vi "Panel Is Dead.vi"(8 "error in (no error)":errorcluster, 11 "Panel Control_Ref in":refnum<class "Panel Controller.lvclass">) -> (0 "error out":errorcluster, 3 "Panel Control_Ref out":refnum<class "Panel Controller.lvclass">)   [LabVIEW 2015, in "Panel Controller.lvclass"]
uses:
  Panel Controller.lvclass
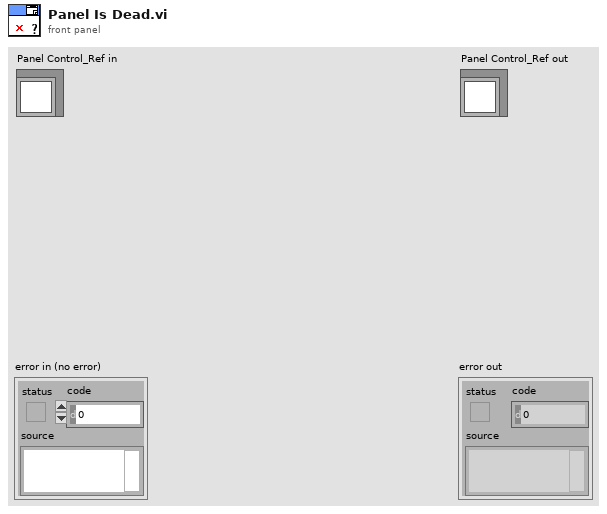
[diagram p1: front panel]
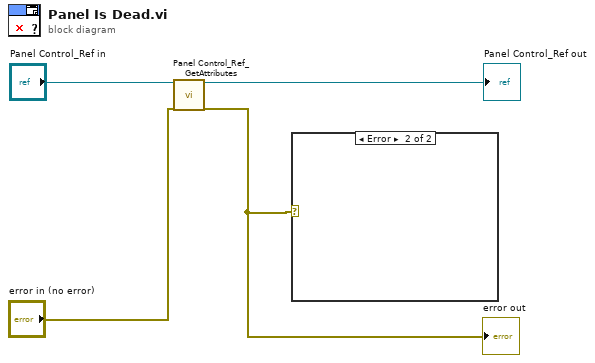
[diagram p0: block diagram]
diagram:
  n1 = call "Panel Control_Ref_GetAttributes.vi"("reference in"="Panel Control_Ref in", "error in (no error)"="error in (no error)") -> ("reference out"=→"Panel Control_Ref out":refnum<class "Panel Controller.lvclass">, "error out"=w1:errorcluster)  [unwired: 14 in, 2 out]
  "error out" <- w1
  n2 = case shown="Error" w1 {
    frame No Error {
    }
    frame Error {
    }
  }
